vi "Find Empty.vi"(11 "Square":refnum<class "Square.lvclass">) -> (2 "Empty Directions":T1[](array[typedef]))   [LabVIEW 2020, in "SquareBattle.lvlib" / "Square.lvclass"]
doc: "Returns an array of all of the directions that contain an empty position and may be safe to move or replicate to. Remember that another square may move into, replicate to, or attack that position so it may end up unsafe due to the actions of other squares.a"
uses:
  Square.lvclass
  Direction.ctl
  Square.lvclass/Square.ctl
  SquareBattle.lvlib
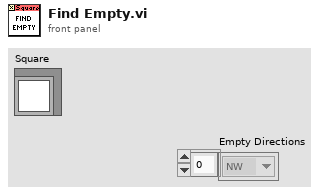
[diagram p1: front panel]
types:
  T1 = typedef "SquareBattle.lvlib/Direction.ctl" = enum16{"NW", "N", "NE", "E", "SE", "S", "SW", "W"}
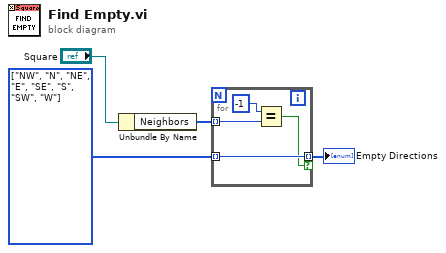
[diagram p0: block diagram]
diagram:
  w2 = T1[] [enum."NW", enum."N", enum."NE", enum."E", enum."SE", enum."S", enum."SW", enum."W"] items=["NW", "N", "NE", "E", "SE", "S", "SW", "W"] ("Enemy Directions")
  n1 = Unbundle By Name("Square") -> ("Neighbors"=w3:i32[])
  n2 = for {
    tunnel: w3 -> [w7] mode=indexing
    tunnel: w2 -> [w8] mode=indexing
    tunnel: [w8] -> w1 mode=indexing if=w6
    n3 = Equal?(x=-1, y=w7) -> (x = y?=w6:bool)
  }
  "Empty Directions" <- w1
